vi "Set command.vi"() -> ()   [LabVIEW 2017]
uses:
  <vilib>/DAQmx/create/channels.llb/DAQmx Create Channel (CO-Pulse Generation-Frequency).vi
  <vilib>/DAQmx/configure/timing.llb/DAQmx Timing (Implicit).vi
  Global/GPIB Numbers.vi
  <instrlib>/Tektronix TDS 200 1000 2000 Series/Public/Data/Read (Single Waveform).vi
  <resource>/objmgr/daqmx.rc
  <instrlib>/Tektronix TDS 200 1000 2000 Series/Tektronix TDS 200 1000 2000 Series.lvlib
panel:
  out "error out":errorcluster
  in  "error in":errorcluster
  in  "Stop":bool
  in  "Counter":tag="Dev1/ctr0"
  in  "Output Terminal":tag="/Dev1/PFI3"
  in  "Set \nVoltage":dbl format="%.6f"
  out "Out of Range":bool
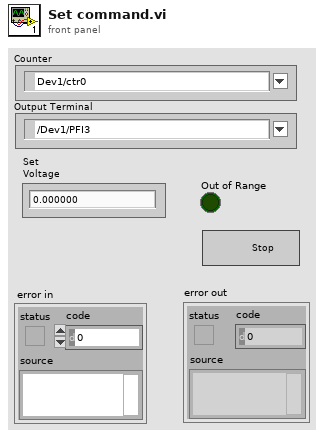
[diagram p1: front panel]
types:
  T1 = typedef "GPIB Type Def.ctl" = cluster{"Name":string, "bus":dbl, "GPIB":dbl, "GPIB as string":string, "byte":i32, "VISA Resource Name":refnum<visa-resource-name>}
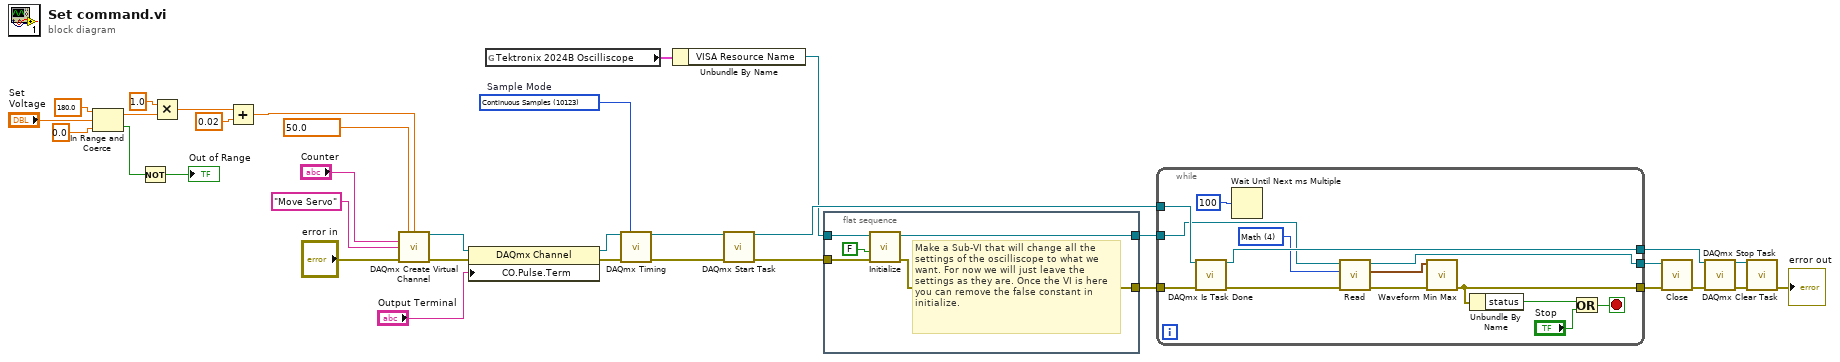
[diagram p0: block diagram]
diagram:
  w12 = 10123 items=["Finite Samples"=10178, "Continuous Samples"=10123, "Hardware Timed Single Point"=12522]  # Sample Mode
  n1 = In Range and Coerce(upper limit=180.0, x="Set \nVoltage", lower limit=0.0) -> (coerced(x)=w22:dbl, In Range?=w24:bool)
  n2 = Not(x=w24) -> (.not. x?=→"Out of Range":bool)
  n3 = Multiply(x=1.0, y=w22) -> (x*y=w20:dbl)
  n4 = Add(x=w20, y=0.02) -> (x+y=w35:dbl)
  n5 = call-poly <vilib>:"DAQmx Create Virtual Channel.vi"("frequency"=50.0 ("Frequency"), "duty cycle"=w35, "counter"="Counter", "name to assign"="Move Servo", "error in"="error in") -> ("task out"=w17:refnum<k21>, "error out"=w16:errorcluster)  [unwired: 9 in]
  n6 = property class="DAQmx Channel"(reference=w17, error in=w16, "CO.Pulse.Term"="Output Terminal") -> (reference out=w33:refnum<k21>, error out=w34:errorcluster)
  n7 = global read "GPIB Numbers.vi" "Tektronix 2024B Oscilliscope"() -> (w6:T1)
  n8 = call-poly <vilib>:"DAQmx Timing.vi"("task/channels in"=w33, "sample mode"=w12, "error in"=w34) -> ("task out"=w32:refnum<k21>, "error out"=w31:errorcluster)  [unwired: 11 in]
  n9 = Unbundle By Name(w6) -> ("VISA Resource Name"=w2:refnum<visa-resource-name>)
  n10 = call <vilib>:"DAQmx Start Task.vi"("task/channels in"=w32, "error in"=w31) -> ("task out"=w11:refnum<k21>, "error out"=w3:errorcluster)  [unwired: 12 in]
  n11 = flat-sequence {
    tunnel: [w38] -> w4
    tunnel: w3 -> [w40]
    tunnel: w2 -> [w39]
    tunnel: [w37] -> w1
    frame #0 {
      # "Make a Sub-VI that will change all the settings of the oscilliscope to what we want. For now we will just leave the settings as they are. Once the VI is here you can remove the false constant in initialize."
      n12 = call <instrlib>:"Initialize.vi"("error in (no error)"=w40, "Reset? (T: Yes)"=FALSE, "VISA resource name"=w39) -> ("error out"=w38:errorcluster, "VISA resource name out"=w37:refnum<visa-resource-name>)  [unwired: 7 in]
    }
  }
  n13 = while {
    tunnel: w11 -> [w54]
    tunnel: w4 -> [w53]
    tunnel: [w45] -> w28
    tunnel: [w44] -> w8
    tunnel: [w46] -> w9
    tunnel: w1 -> [w42]
    stop <- w52 stop-if-true
    w41 = u16 4 items=["Channel 1", "Channel 2", "Channel 3", "Channel 4", "Math", "Reference A", "Reference B", "Reference C", "Reference D", "FFT"] ("Source (0: Channel 1)")
    n14 = call <vilib>:"DAQmx Is Task Done.vi"("task/channels in"=w54, "error in"=w53) -> ("task out"=w45:refnum<k21>, "error out"=w47:errorcluster)  [unwired: 11 in, 1 out]
    n15 = Wait Until Next ms Multiple(millisecond multiple=u32 100) -> ()  [unwired: 1 out]
    n16 = call-poly <instrlib>:"Read.vi"("error in (no error)"=w47, "Source (0: Channel 1)"=w41, "VISA resource name"=w42) -> ("error out"=w48:errorcluster, "Waveform Data"=w43:waveform(dbl), "VISA resource name out"=w46:refnum<visa-resource-name>)  [unwired: 6 in]
    n17 = call <vilib>:"Waveform Min Max.vi"("error in (no error)"=w48, "waveform in"=w43) -> ("error out"=w44:errorcluster)  [unwired: 4 in, 5 out]
    n18 = Unbundle By Name(w44) -> ("status"=w51:bool)
    n19 = Or(x=w51, y="Stop") -> (x .or. y?=w52:bool)
  }
  n20 = call <instrlib>:"Close.vi"("error in (no error)"=w8, "VISA resource name"=w9) -> ("error out"=w7:errorcluster)  [unwired: 9 out]
  n21 = call <vilib>:"DAQmx Stop Task.vi"("task/channels in"=w28, "error in"=w7) -> ("task out"=w30:refnum<k21>, "error out"=w29:errorcluster)  [unwired: 12 in]
  n22 = call <vilib>:"DAQmx Clear Task.vi"("task in"=w30, "error in"=w29) -> ("error out"=→"error out":errorcluster)  [unwired: 13 in]
